vi "Create.vi"(5 "Value":dbl=50.0 format="%#_13g", 9 "Units":T1=enum."dB SPL") -> (8 "Level":refnum<class "Level.lvclass">)   [LabVIEW 2020, in "Level.lvclass"]
uses:
  Level.lvclass
  LevelUnits.ctl
  Level.lvclass/Level.ctl
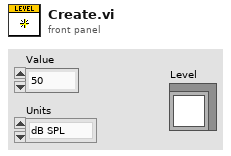
[diagram p1: front panel]
types:
  T1 = typedef "Level.lvclass/LevelUnits.ctl" = enum16{"dB atten", "dB SPL", "dB Vrms", "Volts", "dB mW", "mW", "dB HL", "dB SL"}
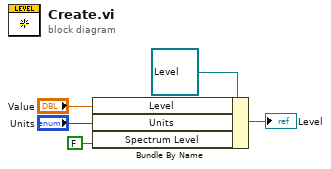
[diagram p0: block diagram]
diagram:
  n1 = Bundle By Name(cluster=refnum<class "Level.lvclass"> refnum ("Level"), "Level"="Value", "Units"="Units", "Spectrum Level"=FALSE ("Serialized.Spectrum Level")) -> (→"Level":refnum<class "Level.lvclass">)
